vi "Problem 2.vi"() -> ()   [LabVIEW 2025]
panel:
  out "7 Digit Floating Points":dbl format="%#_7f"
  out "6 Digit Floating Points (Default)":dbl format="%#_6f"
  out "Norm Sum (Correct)":i32
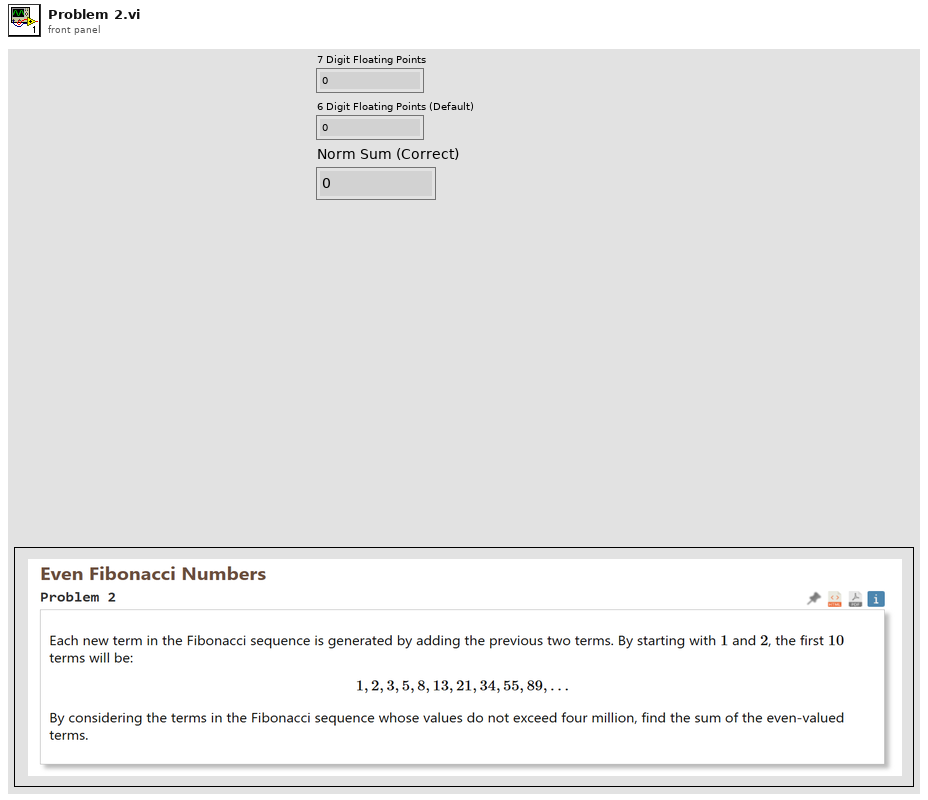
[diagram p1: front panel]
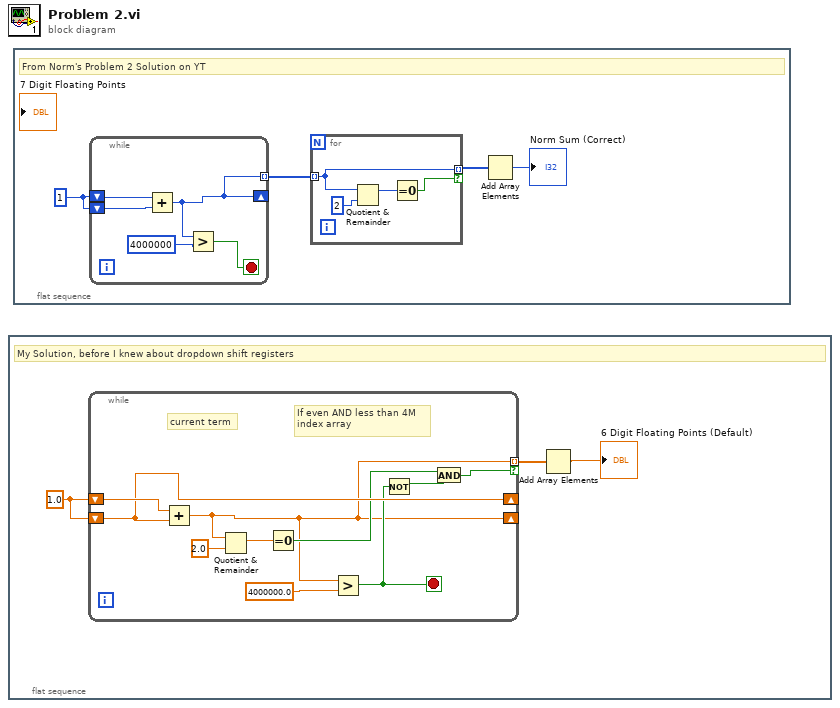
[diagram p0: block diagram]
diagram:
  n1 = flat-sequence {
    frame #0 {
      w1 = 1.0
      # "My Solution, before I knew about dropdown shift registers"
      n2 = while {
        shift-right: [w12] -> _
        shift-left: w1 -> [w13]
        shift-right: [w4] -> _
        shift-left: w1 -> [w12]
        tunnel: [w4] -> w3 mode=indexing if=w7
        stop <- w6 stop-if-true
        # "If even AND less than 4M\nindex array"
        # "current term"
        n3 = Add(x=w13, y=w12) -> (x+y=w4:dbl)
        n4 = Quotient & Remainder(x=w4, y=2.0) -> (x-y*floor(x/y)=w10:dbl)  [unwired: 1 out]
        n5 = Equal To 0?(x=w10) -> (x = 0?=w9:bool)
        n6 = Greater?(x=w4, y=4000000.0) -> (0:w6:bool)
        n7 = Not(x=w6) -> (.not. x?=w5:bool)
        n8 = And(x=w9, y=w5) -> (x .and. y?=w7:bool)
      }
      n9 = Add Array Elements(numeric array=w3) -> (sum=→"6 Digit Floating Points (Default)":dbl)
    }
  }
  n10 = flat-sequence {
    frame #0 {
      w17 = 1
      # "From Norm's Problem 2 Solution on YT"
      n11 = while {
        shift-right: [w22] -> _
        shift-left: w17 -> [w26]
        shift-left: w17 -> [w25]
        tunnel: [w22] -> w16 mode=indexing
        stop <- w23 stop-if-true
        n12 = Add(x=w26, y=w25) -> (x+y=w22:i32)
        n13 = Greater?(x=w22, y=4000000) -> (0:w23:bool)
      }
      n14 = for {
        tunnel: w16 -> [w19] mode=indexing
        tunnel: [w19] -> w15 mode=indexing if=w18
        n15 = Quotient & Remainder(x=w19, y=2) -> (x-y*floor(x/y)=w20:i32)  [unwired: 1 out]
        n16 = Equal To 0?(x=w20) -> (x = 0?=w18:bool)
      }
      n17 = Add Array Elements(numeric array=w15) -> (sum=→"Norm Sum (Correct)":i32)
    }
  }
